vi "PrintFrames.vi"(6 "Path":path=path "C:/LabViewTesty", 7 "Frame":cluster{i32[], i32[]}[](graph), 8 "In":cluster{i32[], i32[]}(graph), 9 "Nak":cluster{i32[], i32[]}(graph), 10 "Out":cluster{i32[], i32[]}(graph)) -> ()   [LabVIEW 2014]
panel:
  out "Frames":T1
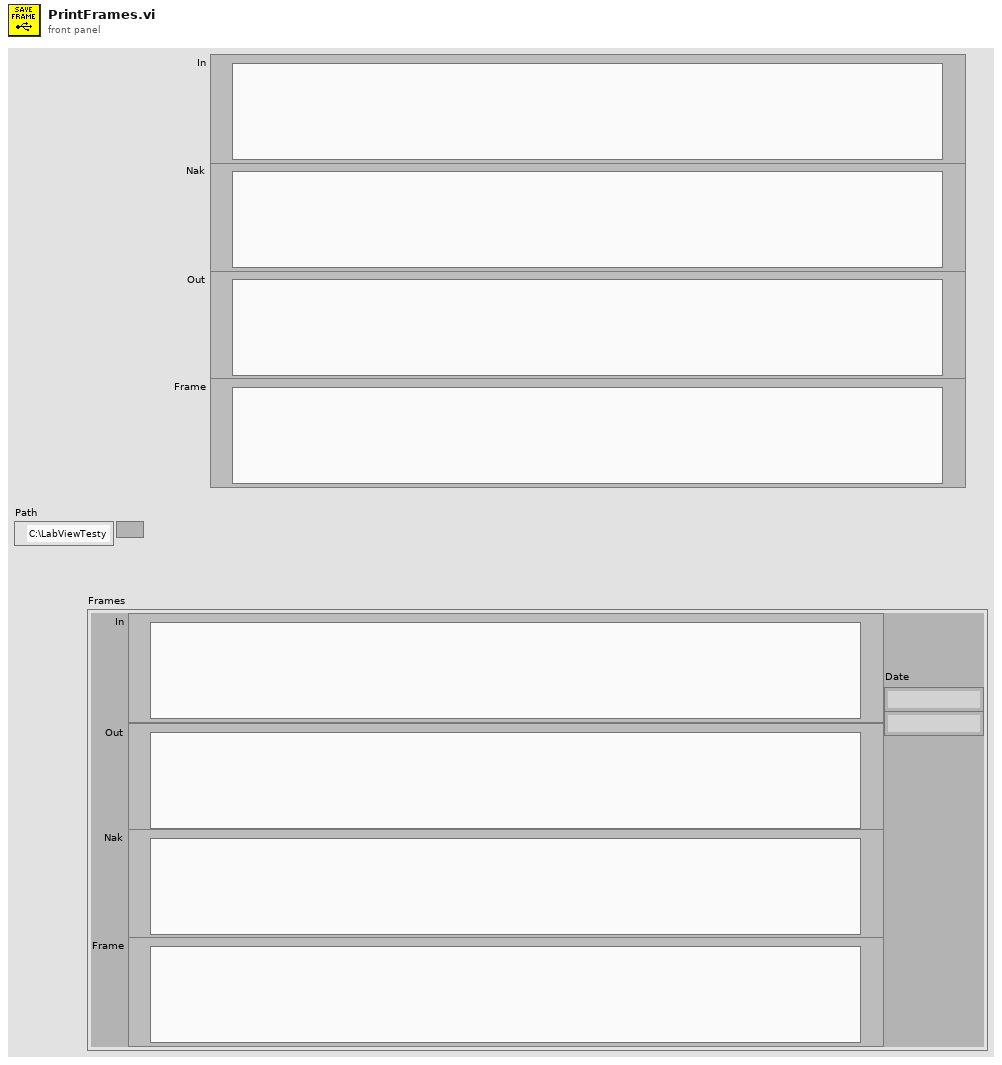
[diagram p1: front panel]
types:
  T1 = cluster{"In":cluster{i32[], i32[]}, "Out":cluster{i32[], i32[]}, "Nak":cluster{i32[], i32[]}, "Frame":cluster{i32[], i32[]}[], "Date":string, "String 2":string}
  T2 = typedef "imagedata.ctl" = cluster{"image type":i32, "image depth":i32, "image":u8[], "mask":u8[], "colors":u32[], "Rectangle":cluster{"left":i16, "top":i16, "right":i16, "bottom":i16}}
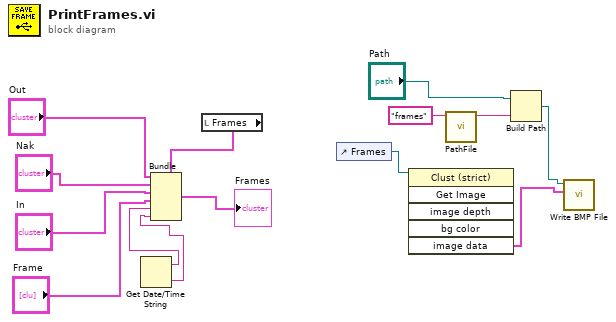
[diagram p0: block diagram]
diagram:
  n1 = Get Date/Time String() -> (date string=w7:string, time string=w6:string)  [unwired: 3 in]
  n2 = local read "Frames"() -> (w10:T1)
  n3 = Bundle(cluster=w10, "In"="Out", "Out"="Nak", "Nak"="In", "Frame"="Frame", "Date"=w7, "String 2"=w6) -> (→"Frames":T1)
  n4 = control-ref of="Frames"() -> (w8:refnum<vi>)
  n5 = invoke class="Clust (strict)" method="Get Image"(reference=w8) -> ("image data"=w5:T2)  [unwired: 5 in, 5 out]
  n6 = call "PathFile.vi"("NameFile"="frames") -> ("stringNameFile"=w1:string)  [unwired: 10 in]
  n7 = Build Path(base path="Path", name or relative path=w1) -> (appended path=w4:path)
  n8 = call <vilib>:"Write BMP File.vi"("image data"=w5, "path to BMP file"=w4) -> ()  [unwired: 8 in, 2 out]
